vi "Main.vi"() -> ()   [LabVIEW 2012]
uses:
  Consumer Message.ctl
panel:
  out "待执行状态":string
  out "高优先级？":bool
  out "积压空间":u8(slide) scale=0.0..100.0
  out "已处理值":i32
  in  "高优先级消息":bool
  in  "标准优先级消息":bool
  in  "停止":bool
  # "待入队处理的\n消息数量"
  # "消费者循环中\n当前正在处理的数据"
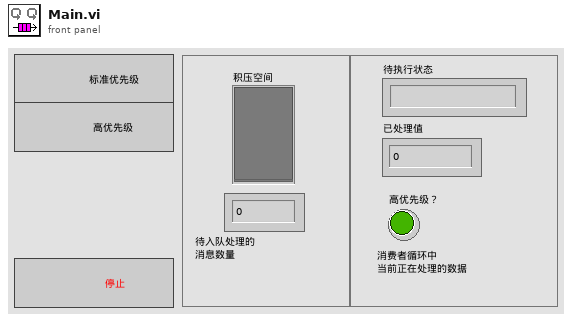
[diagram p1: front panel]
types:
  T1 = typedef "Consumer Message.ctl" = cluster{"消费者状态":string, "布尔数据":bool, "数值数据":i32}
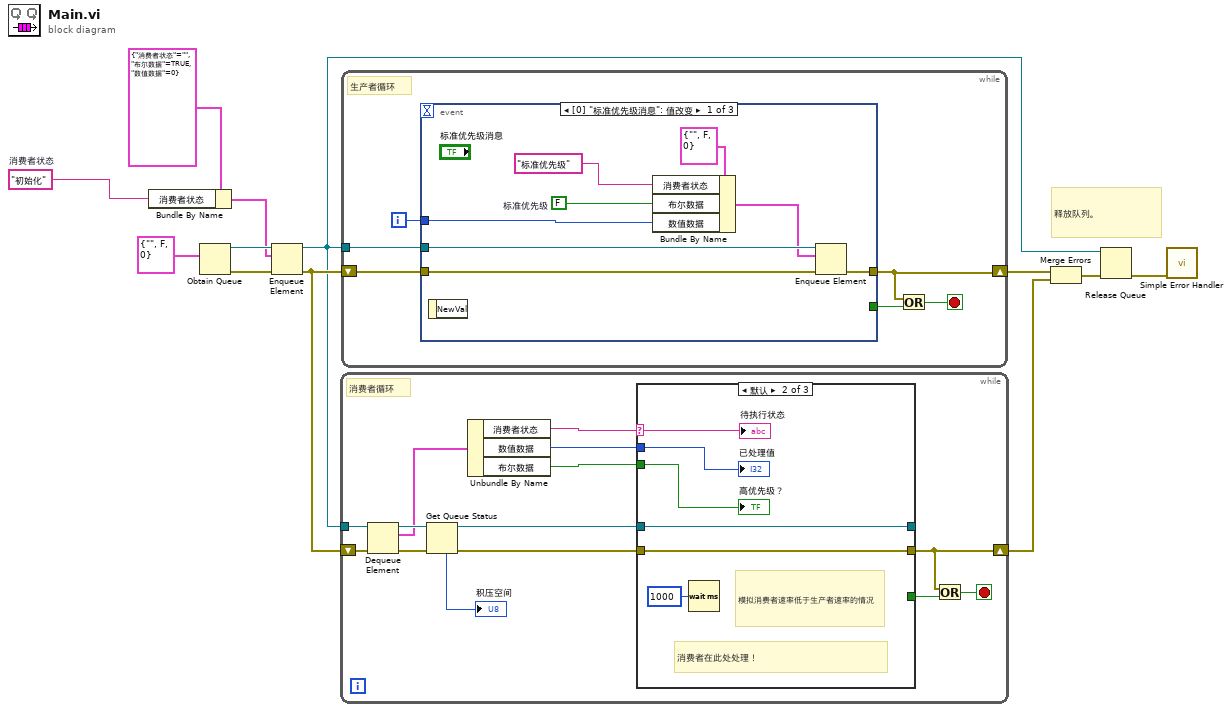
[diagram p0: block diagram]
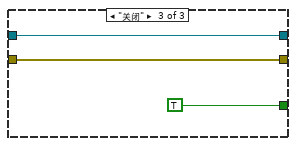
[diagram p3: hidden frame]
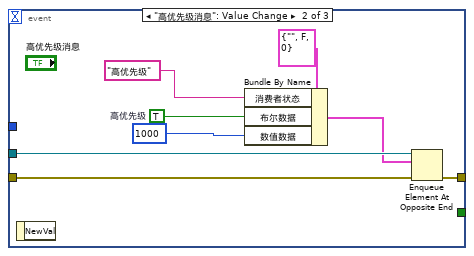
[diagram p4: hidden frame]
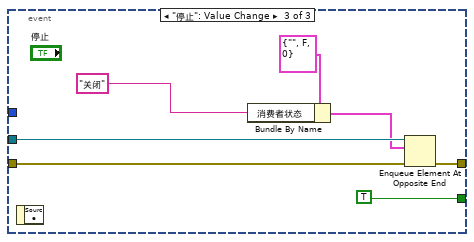
[diagram p5: hidden frame]
diagram:
  w1 = "初始化"  # 消费者状态
  # "释放队列。"
  n1 = Bundle By Name ("按名称捆绑")(cluster=T1 {"消费者状态"="", "布尔数据"=TRUE, "数值数据"=0} ("消费者消息"), "消费者状态"=w1) -> (w2:T1)
  n2 = Obtain Queue ("获取队列引用")(element data type=T1 {"消费者状态"="", "布尔数据"=FALSE, "数值数据"=0}) -> (queue out=w6:refnum<queue>, error out=w12:errorcluster)  [unwired: 4 in, 1 out]
  n3 = Enqueue Element ("元素入队列")(queue=w6, element=w2, error in (no error)=w12) -> (queue out=w5:refnum<queue>, error out=w7:errorcluster)  [unwired: 1 in, 1 out]
  n4 = while {
    tunnel: w5 -> [w24]
    shift-right: [w13] -> w11
    shift-left: w7 -> [w23]
    stop <- w14 stop-if-true
    # "消费者循环"
    n5 = Dequeue Element ("元素出队列")(queue=w24, error in (no error)=w23) -> (queue out=w25:refnum<queue>, element=w22:T1, error out=w26:errorcluster)  [unwired: 1 in, 1 out]
    n6 = Get Queue Status ("获取队列状态")(queue=w25, error in (no error)=w26) -> (queue out=w16:refnum<queue>, error out=w20:errorcluster, # elements in queue=→"积压空间":i32)  [unwired: 1 in, 5 out]
    n7 = Unbundle By Name ("按名称解除捆绑")(w22) -> ("消费者状态"=w21:string, "数值数据"=w19:i32, "布尔数据"=w17:bool)
    n8 = case shown="默认" w21 {
      selector: w21 -> [_ w31 _]
      tunnel: [_ _ TRUE] -> w15
      tunnel: w20 -> [w27 w29 w35]
      tunnel: [w27 w29 w35] -> w13
      tunnel: w19 -> [_ w34 _]
      tunnel: w17 -> [_ w33 _]
      tunnel: w16 -> [w28 w32 w36]
      tunnel: [w28 w32 w36] -> _
      frame "初始化" {
      }
      frame Default {
        # "模拟消费者速率低于生产者速率的情况"
        # "消费者在此处处理！"
        n9 = Wait (ms) ("等待(ms)")(milliseconds to wait=u32 1000 ("等待时间（毫秒）")) -> ()  [unwired: 1 out]
        "已处理值" <- w34
        "高优先级？" <- w33
        "待执行状态" <- w31
      }
      frame "关闭" {
      }
    }
    n10 = Or ("或")(x=w13, y=w15) -> (x .or. y?=w14:bool)
  }
  n11 = while {
    shift-right: [w38] -> w10
    shift-left: w7 -> [w42]
    tunnel: w5 -> [w43]
    i -> [w41]
    stop <- w39 stop-if-true
    # "生产者循环"
    n12 = event shown="[0] \"标准优先级消息\": 值改变" {
      selector: _ -> [_ _ _]
      dyn-events: _ -> [_ _ _]
      timeout: _ -> [_ _ _]
      tunnel: w43 -> [w51 w58 w66]
      tunnel: w42 -> [w49 w57 w64]
      tunnel: [w50 w59 w63] -> w38
      tunnel: [_ _ TRUE] -> w40
      tunnel: w41 -> [w48 _ _]
      event "标准优先级消息": Value Change {
        w45 = FALSE  # 标准优先级
        n13 = event-data ("事件数据节点")() -> ()  [unwired: 1 in, 1 out]
        n14 = Bundle By Name ("按名称捆绑")(cluster=T1 {"消费者状态"="", "布尔数据"=FALSE, "数值数据"=0}, "消费者状态"="标准优先级" ("字符串数据"), "布尔数据"=w45, "数值数据"=w48) -> (w47:T1)
        n15 = Enqueue Element ("元素入队列")(queue=w51, element=w47, error in (no error)=w49) -> (error out=w50:errorcluster)  [unwired: 1 in, 2 out]
      }
      event "高优先级消息": Value Change {
        w53 = TRUE  # 高优先级
        n16 = event-data ("事件数据节点")() -> ()  [unwired: 1 in, 1 out]
        n17 = Bundle By Name ("按名称捆绑")(cluster=T1 {"消费者状态"="", "布尔数据"=FALSE, "数值数据"=0}, "消费者状态"="高优先级" ("字符串数据"), "布尔数据"=w53, "数值数据"=1000) -> (w55:T1)
        n18 = Enqueue Element At Opposite End ("队列最前端插入元素")(queue=w58, element=w55, error in (no error)=w57) -> (error out=w59:errorcluster)  [unwired: 1 in, 2 out]
      }
      event "停止": Value Change {
        n19 = event-data ("事件数据节点")() -> ()  [unwired: 1 in, 1 out]
        n20 = Bundle By Name ("按名称捆绑")(cluster=T1 {"消费者状态"="", "布尔数据"=FALSE, "数值数据"=0}, "消费者状态"="关闭") -> (w60:T1)
        n21 = Enqueue Element At Opposite End ("队列最前端插入元素")(queue=w66, element=w60, error in (no error)=w64) -> (error out=w63:errorcluster)  [unwired: 1 in, 2 out]
      }
    }
    n22 = Or ("或")(x=w38, y=w40) -> (x .or. y?=w39:bool)
  }
  n23 = Merge Errors ("合并错误")(w10, w11) -> (w9:errorcluster)
  n24 = Release Queue ("释放队列引用")(queue=w5, error in (no error)=w9) -> (error out=w4:errorcluster)  [unwired: 1 in, 2 out]
  n25 = call <vilib>:"Simple Error Handler.vi"("error in (no error)"=w4) -> ()  [unwired: 4 in, 5 out]
